vi "Thermometer.vi"(1 "Temp Scale":bool) -> (0 "Temperature":dbl(slide) scale=0.0..100.0)   [LabVIEW 2011]
doc: "This VI is the solution to an exercise in the LabVIEW Core I course.\n\nIt measures temperature using the temperature sensor on the DAQ Signal Accessory."
uses:
  Instance           1 19Saved   Thermometer .vi
  Instance           2 19Saved   Thermometer .vi
panel:
  # "deg C"
  # "deg F"
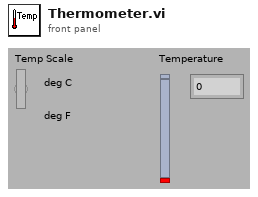
[diagram p1: front panel]
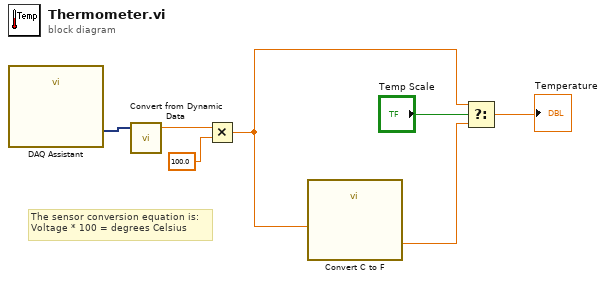
[diagram p0: block diagram]
diagram:
  # "The sensor conversion equation is: \nVoltage * 100 = degrees Celsius"
  n1 = call "DAQ Assistant"() -> ("data"=w4:dynamicdata)  [unwired: 17 in, 2 out]
  n2 = call "Convert from Dynamic Data"("Dynamic Data Type"=w4) -> ("Scalar"=w2:dbl)  [unwired: 3 in]
  n3 = Multiply(x=w2, y=100.0) -> (x*y=w3:dbl)
  n4 = call "Convert C to F.vi"("deg C"=w3) -> ("deg F"=w6:dbl)
  n5 = Select(t=w3, s="Temp Scale", f=w6) -> (s? t:f=→"Temperature":dbl)
